vi "Recurse Path.vi"(9 "Next Cave":i32, 10 "Parent Path":T1, 11 "Cave System In":T2) -> (2 "Found Paths":T1[](array[typedef]))   [LabVIEW 2020]
uses:
  Cave System.ctl
  Cave.ctl
  Path.ctl
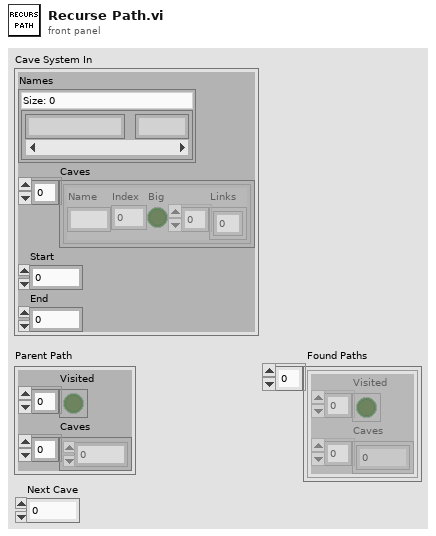
[diagram p1: front panel]
types:
  T1 = typedef "Path.ctl" = cluster{"Visited":bool[], "Caves":i32[]}
  T2 = typedef "Cave System.ctl" = cluster{"Names":map{string, i32}, "Caves":T3[], "Start":i32, "End":i32}
  T3 = typedef "Cave.ctl" = cluster{"Name":string, "Index":i32, "Big":bool, "Links":i32[]}
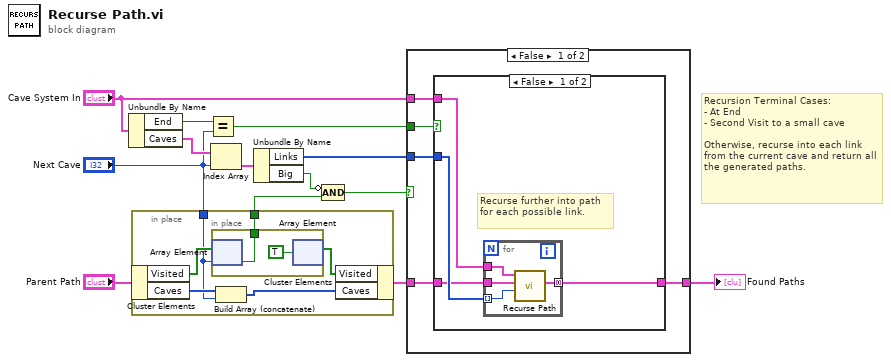
[diagram p0: block diagram]
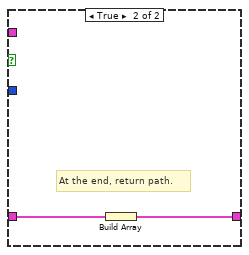
[diagram p2: hidden frame]
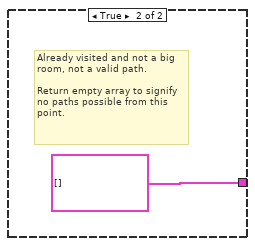
[diagram p3: hidden frame]
diagram:
  # "Recursion Terminal Cases:\n- At End\n- Second Visit to a small cave\n\nOtherwise, recurse into each link from the current cave and return all the generated paths."
  n1 = Unbundle By Name("Cave System In") -> ("End"=w3:i32, "Caves"=w12:T3[])
  n2 = in-place {
    in-place-border: [w18] -> w9
    in-place-border: "Next Cave" -> [w16]
    n3 = in-place-cluster #1("Parent Path") -> ("Visited"=w19:bool[], "Caves"=w17:i32[])
    n4 = in-place {
      in-place-border: [w21] -> w18
      n5 = in-place-array #2(w19, w16) -> (w21:bool)
      n6 = in-place-array #2(TRUE ("element")) -> (w14:bool[])  [unwired: 1 out]
    }
    n7 = Build Array (concatenate)(w17, w16) -> (w15:i32[])
    n8 = in-place-cluster #1("Visited"=w14, "Caves"=w15) -> (w8:T1)
  }
  n9 = Equal?(x=w3, y="Next Cave") -> (x = y?=w2:bool)
  n10 = Index Array(array=w12, index="Next Cave") -> (element=w11:T3)
  n11 = Unbundle By Name(w11) -> ("Links"=w6:i32[], "Big"=w10:bool)
  n12 = Compound Arithmetic op=AND(invert w10, w9) -> (w7:bool)
  n13 = case shown="False" w7 {
    tunnel: w8 -> [w25 _]
    tunnel: w6 -> [w23 _]
    tunnel: [w24 T1[] [] ("Found Paths")] -> w5
    tunnel: w2 -> [w26 _]
    tunnel: "Cave System In" -> [w22 _]
    frame False {
      n14 = case shown="False" w26 {
        tunnel: w25 -> [w29 w36]
        tunnel: [w28 w35] -> w24
        tunnel: w23 -> [w30 _]
        tunnel: w22 -> [w27 _]
        frame False {
          # "Recurse further into path for each possible link."
          n15 = for {
            tunnel: w30 -> [w34] mode=indexing
            tunnel: w29 -> [w33]
            tunnel: [w32] -> w28 mode=concatenating
            tunnel: w27 -> [w31]
            n16 = call "Recurse Path.vi"("Next Cave"=w34, "Parent Path"=w33, "Cave System In"=w31) -> ("Found Paths"=w32:T1[])  [unwired: 8 in]
          }
        }
        frame True {
          # "At the end, return path."
          n17 = Build Array(w36) -> (w35:T1[])
        }
      }
    }
    frame True {
      # "Already visited and not a big room, not a valid path.\n\nReturn empty array to signify no paths possible from this point."
    }
  }
  "Found Paths" <- w5
